vi "Convert Timestamp to JSON Citadel Timestamp.vi"(11 "time stamp":timestamp) -> (3 "Citadel date/time string":string)   [LabVIEW 2019]
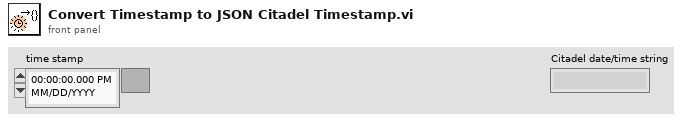
[diagram p1: front panel]
types:
  T1 = typedef "LVDateTimeRec.ctl" = cluster{"fractional second":dbl, "second":i32, "minute":i32, "hour":i32, "day of month":i32, "month":i32, "year":i32, "day of week":i32, "day of year":i32, "DST":i32}
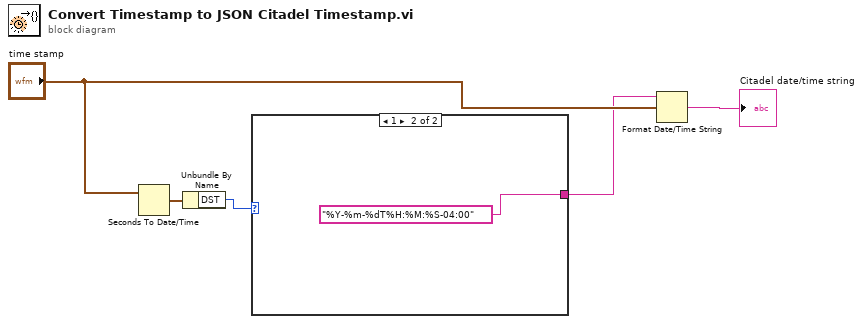
[diagram p0: block diagram]
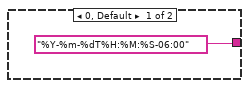
[diagram p2: hidden frame]
diagram:
  n1 = Seconds To Date/Time(time stamp (now)="time stamp") -> (date time rec=w3:T1)  [unwired: 1 in]
  n2 = Unbundle By Name(w3) -> ("DST"=w2:i32)
  n3 = case shown="1" w2 {
    tunnel: ["%Y-%m-%dT%H:%M:%S-06:00" ("time format string (%c)") "%Y-%m-%dT%H:%M:%S-04:00" ("time format string (%c)")] -> w1
    frame 0, Default {
    }
    frame 1 {
    }
  }
  n4 = Format Date/Time String(time format string (%c)=w1, seconds (now)="time stamp") -> (date/time string=→"Citadel date/time string":string)  [unwired: 1 in]
